vi "Error Handler Dialog.vi"(7 "NoContinue (F)":bool, 11 "ErrorText":string="This is a test error message.") -> (1 "TerminateApp?":bool, 2 "DisableDialog?":bool, 3 "Shutdown?":bool)   [LabVIEW 2017, in "ErrorHandler.lvclass"]
doc: "Developed by Kevin Thompson\nkevin@thompsonengineering.net\n\nCopyright 2018\nThompson Engineering, LLC"
uses:
  ErrorHandler.lvclass
panel:
  in  "TerminateApp":bool
  in  "DisableDialog":bool
  in  "Shutdown":bool
  in  "Continue":bool
  # "[ESC]"
  # "[RETURN]"
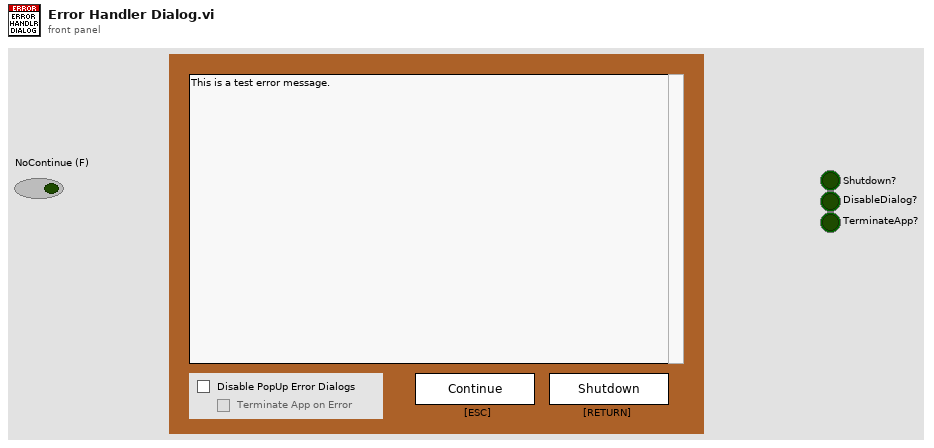
[diagram p1: front panel]
types:
  T1 = enum8{"Enabled", "Disabled", "Disabled and Grayed Out"}
  T2 = enum32{"Invalid", "Default", "Floating", "Floating/Auto-Hide", "Modal"}
  T3 = enum32{"Invalid", "Standard", "Closed", "Hidden", "Minimized", "Maximized"}
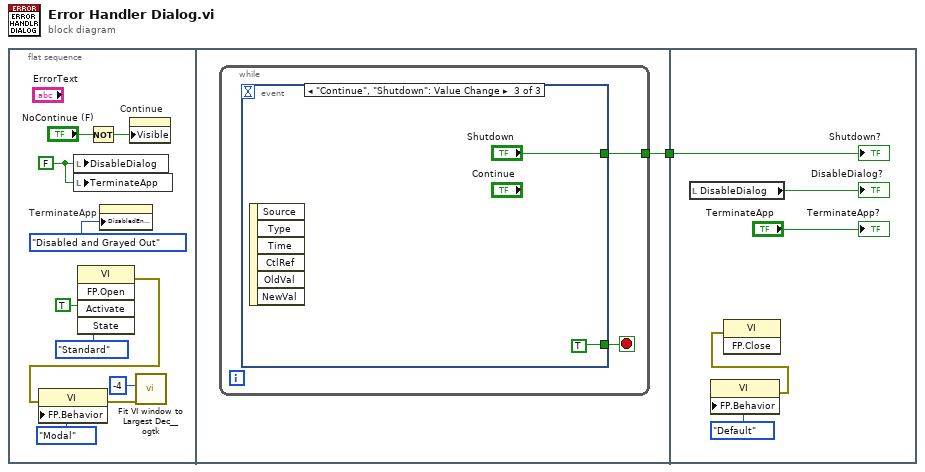
[diagram p0: block diagram]
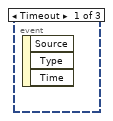
[diagram p2: hidden frame]
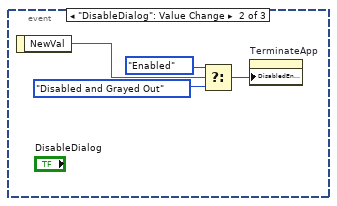
[diagram p3: hidden frame]
diagram:
  n1 = flat-sequence {
    tunnel: [w12] -> w1
    tunnel: w1 -> [w22]
    frame #0 {
      w3 = FALSE
      n2 = local write "DisableDialog"(w3) -> ()
      n3 = local write "TerminateApp"(w3) -> ()
      n4 = invoke class="VI" method="FP.Open"("Activate"=TRUE ("Activate?"), "State"=T3."Standard") -> (error out=w8:errorcluster)  [unwired: 3 in, 4 out]
      n5 = property class="VI"(error in=w8, "FP.Behavior"=T2."Modal" ("Front Panel Window:Behavior")) -> (error out=w7:errorcluster)  [unwired: 1 in, 1 out]
      n6 = Not(x="NoContinue (F)") -> (.not. x?=w4:bool)
      n7 = property on="TerminateApp" class="Bool (strict)"("DisabledEnum"=T1."Disabled and Grayed Out" ("Disabled")) -> ()  [unwired: 2 in, 2 out]
      n8 = property on="Continue" class="Bool"("Visible"=w4) -> ()  [unwired: 2 in, 2 out]
      n9 = call <userlib>:"Fit VI window to Largest Dec__ogtk.vi"("error in (no error)"=w7, "border spacing (2 px)"=-4) -> ()  [unwired: 4 in, 2 out]
    }
    frame #1 {
      n10 = while {
        tunnel: [w13] -> w12
        stop <- w14 stop-if-true
        n11 = event shown="[2] \"Continue\", \"Shutdown\": Value Change" {
          selector: _ -> [_ _ _]
          dyn-events: _ -> [_ _ _]
          timeout: _ -> [_ _ _]
          tunnel: [_ _ TRUE] -> w14
          tunnel: [_ _ "Shutdown"] -> w13
          event Timeout {
            n12 = event-data() -> ()  [unwired: 1 in, 3 out]
          }
          event "DisableDialog": Value Change {
            n13 = event-data() -> ("NewVal"=w15:bool)  [unwired: 1 in]
            n14 = Select(t=T1."Enabled" ("Disabled"), s=w15, f=T1."Disabled and Grayed Out" ("Disabled")) -> (s? t:f=w17:T1)
            n15 = property on="TerminateApp" class="Bool (strict)"("DisabledEnum"=w17) -> ()  [unwired: 2 in, 2 out]
          }
          event "Continue", "Shutdown": Value Change {
            n16 = event-data() -> ()  [unwired: 1 in, 6 out]
          }
        }
      }
    }
    frame #2 {
      n17 = local read "DisableDialog"() -> (→"DisableDialog?":bool)
      n18 = property class="VI"("FP.Behavior"=T2."Default" ("Front Panel Window:Behavior")) -> (error out=w24:errorcluster)  [unwired: 2 in, 1 out]
      n19 = invoke class="VI" method="FP.Close"(error in=w24) -> ()  [unwired: 2 in, 3 out]
      "Shutdown?" <- w22
      "TerminateApp?" <- "TerminateApp"
    }
  }
